vi "replaceNode.vi"(8 "error in (no error)":errorcluster, 10 "ReplacerNode":refnum<class "xceNode.lvclass">, 11 "ReplaceNode":refnum<class "xceNode.lvclass">) -> (0 "error out":errorcluster, 2 "ReplacerNode out":refnum<class "xceNode.lvclass">, 3 "ReplaceNode out":refnum<class "xceNode.lvclass">)   [LabVIEW 2013, in "xceNode.lvclass"]
doc: "Replaces one nodes location in the tree data structure with another node. Used primarily to swap object in/out of a tree data structure."
uses:
  xceNode.lvclass
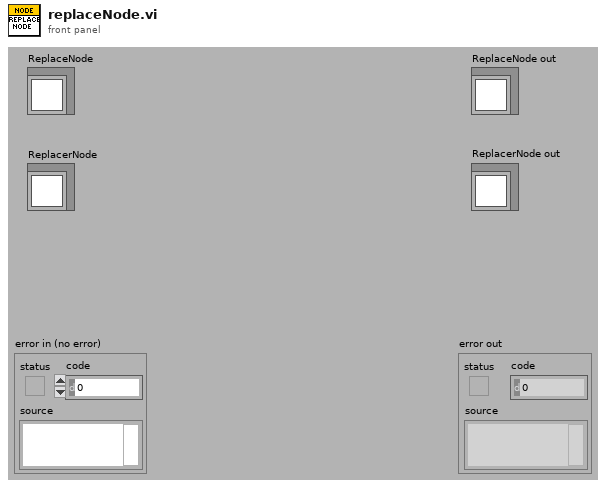
[diagram p1: front panel]
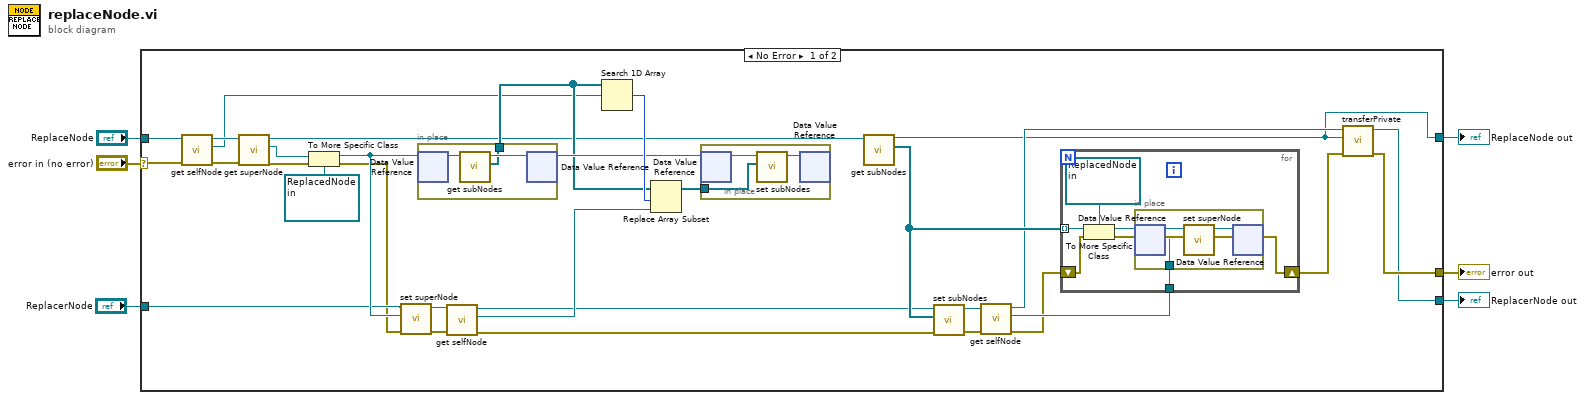
[diagram p0: block diagram]
diagram:
  n1 = case shown="No Error" "error in (no error)" {
    selector: "error in (no error)" -> [w25 w55]
    tunnel: [w10 w55] -> w5
    tunnel: "ReplacerNode" -> [w28 w53]
    tunnel: "ReplaceNode" -> [w26 w54]
    tunnel: [w8 w54] -> w2
    tunnel: [w7 w53] -> w1
    frame No Error {
      n2 = call "get selfNode.vi"("error in (no error)"=w25, "xceNode in"=w26) -> ("error out"=w24:errorcluster, "selfNode*"=w23:refnum<data-value>, "xceNode out"=w27:refnum<class "xceNode.lvclass">)  [unwired: 7 in]
      n3 = call "get superNode.vi"("error in (no error)"=w24, "xceNode in"=w27) -> ("error out"=w37:errorcluster, "superNode*"=w34:refnum<data-value>, "xceNode out"=w19:refnum<class "xceNode.lvclass">)  [unwired: 7 in]
      n4 = To More Specific Class(target class=refnum<data-value> refnum ("ReplacerNode* in"), reference=w34, error in=w37) -> (specific class reference=w35:refnum<data-value>, error out=w16:errorcluster)
      n5 = call "set superNode.vi"("error in (no error)"=w16, "superNode*"=w35, "xceNode in"=w28) -> ("error out"=w22:errorcluster, "xceNode out"=w21:refnum<class "xceNode.lvclass">)  [unwired: 7 in]
      n6 = in-place {
        in-place-border: [w50] -> w29
        n7 = in-place-dvr #1(w35) -> (w52:refnum<class "xceNode.lvclass">)  [unwired: 1 out]
        n8 = call "get subNodes.vi"("xceNode in"=w52) -> ("subNodes[]*"=w50:refnum<data-value>[], "xceNode out"=w51:refnum<class "xceNode.lvclass">)  [unwired: 8 in, 1 out]
        n9 = in-place-dvr #1(w51) -> (w32:refnum<data-value>)  [unwired: 1 out]
      }
      n10 = call "get selfNode.vi"("error in (no error)"=w22, "xceNode in"=w21) -> ("error out"=w17:errorcluster, "selfNode*"=w20:refnum<data-value>, "xceNode out"=w18:refnum<class "xceNode.lvclass">)  [unwired: 7 in]
      n11 = Search 1D Array(1D array=w29, element=w23) -> (index of element=w33:i32)  [unwired: 1 in]
      n12 = Replace Array Subset(array=w29, new element=w20, index=w33) -> (w31:refnum<data-value>[])
      n13 = in-place {
        in-place-border: w31 -> [w47]
        n14 = in-place-dvr #2(w32) -> (w49:refnum<class "xceNode.lvclass">)  [unwired: 1 out]
        n15 = call "set subNodes.vi"("subNodes[]*"=w47, "xceNode in"=w49) -> ("xceNode out"=w48:refnum<class "xceNode.lvclass">)  [unwired: 8 in, 1 out]
        n16 = in-place-dvr #2(w48) -> ()  [unwired: 2 out]
      }
      n17 = call "get subNodes.vi"("xceNode in"=w19) -> ("subNodes[]*"=w30:refnum<data-value>[], "xceNode out"=w8:refnum<class "xceNode.lvclass">)  [unwired: 8 in, 1 out]
      n18 = call "set subNodes.vi"("error in (no error)"=w17, "subNodes[]*"=w30, "xceNode in"=w18) -> ("error out"=w14:errorcluster, "xceNode out"=w15:refnum<class "xceNode.lvclass">)  [unwired: 7 in]
      n19 = call "get selfNode.vi"("error in (no error)"=w14, "xceNode in"=w15) -> ("error out"=w12:errorcluster, "selfNode*"=w13:refnum<data-value>, "xceNode out"=w9:refnum<class "xceNode.lvclass">)  [unwired: 7 in]
      n20 = for {
        tunnel: w30 -> [w43] mode=indexing
        tunnel: w13 -> [w39]
        shift-right: [w40] -> w11
        shift-left: w12 -> [w38]
        n21 = To More Specific Class(target class=refnum<data-value> refnum ("ReplacerNode* in"), reference=w43, error in=w38) -> (specific class reference=w41:refnum<data-value>, error out=w40:errorcluster)
        n22 = in-place {
          in-place-border: w39 -> [w44]
          n23 = in-place-dvr #3(w41) -> (w46:refnum<class "xceNode.lvclass">)  [unwired: 1 out]
          n24 = call "set superNode.vi"("superNode*"=w44, "xceNode in"=w46) -> ("xceNode out"=w45:refnum<class "xceNode.lvclass">)  [unwired: 8 in, 1 out]
          n25 = in-place-dvr #3(w45) -> ()  [unwired: 2 out]
        }
      }
      n26 = call-dynamic "transferPrivate.vi"("error in (no error)"=w11, "TransferFrom in"=w8, "TransferTo in"=w9) -> ("error out"=w10:errorcluster, "TransferTo out"=w7:refnum<class "xceNode.lvclass">)  [unwired: 6 in, 1 out]
    }
    frame Error {
    }
  }
  "error out" <- w5
  "ReplaceNode out" <- w2
  "ReplacerNode out" <- w1
